vi "Main.vi"(8 "error in":errorcluster, 11 "Registration in":refnum<class "Registration.lvclass">) -> (0 "error out":errorcluster, 3 "Registration out":refnum<class "Registration.lvclass">)   [LabVIEW 2023, in "Registration.lvclass"]
doc: "The <b>Queued Message Handler</b> of the Worker that owns this VI."
uses:
  Registration.lvclass
  C:/Program Files/National Instruments/LabVIEW 2023/vi.lib/addons/_Workers/Library/Classes/Worker/Worker.lvclass
  rqp_Data.ctl
  Initialization Data.ctl
  Response Cases.ctl
  Registration.lvclass/Registration.ctl
  rql_Set File Path.ctl
  rqp_Start.ctl
  <vilib>/Utility/sysdir.llb/System Directory Type.ctl
  <vilib>/addons/_Workers/Library/Case Label.ctl
  rqp_Timeout.ctl
  <vilib>/Utility/file.llb/Write Delimited Spreadsheet (string).vi
  <vilib>/Utility/error.llb/Error Cluster From Error Code.vi
  <vilib>/addons/_Workers/Library/Classes/Message Queue/Message Queue.lvclass
  <vilib>/ErrorRing/Error Ring.xnode
  <vilib>/addons/_Workers/Library/Workers.lvlib
  Work Planer/Work Planer.lvclass
  C:/Program Files/National Instruments/LabVIEW 2023/vi.lib/addons/_Workers/Library/Classes/Workers Object/Workers Object.lvclass
  J:/Work/Cortech/KTM 1001/Workers/Registration Worker/Registration.lvclass
panel:
  in  "Period, s":u32 caption="Период регистрации, сек"
  in  "set_path":bool
  in  "open_F":bool
  in  "Registr start":bool
  out "file_path":string caption="Файл регистрации"
  out "Таймаут":u32
  out "Data":T1 {"Уд. сопротивление" format="%#.3f"; "Сопротивление" format="%#.3f"; "Диаметр" format="%#.3f"; "Длина" format="%#.3f"}
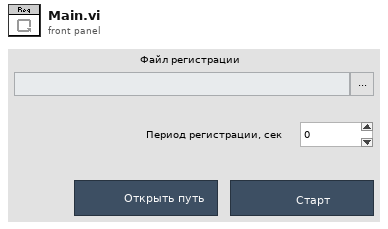
[diagram p1: front panel]
types:
  T1 = typedef "Registration.lvclass/rqp_Data.ctl" = cluster{"Дата":string, "Время":string, "Длина":dbl, "Диаметр":dbl, "Сопротивление":dbl, "Уд. сопротивление":dbl}
  T2 = typedef "Registration.lvclass/rql_Set File Path.ctl" = cluster{"String":string}
  T3 = enum8{"Enabled", "Disabled", "Disabled and Grayed Out"}
  T4 = typedef "Registration.lvclass/rqp_Start.ctl" = cluster{"Start":bool}
  T5 = typedef "Registration.lvclass/rqp_Timeout.ctl" = cluster{"Таймаут":u32}
  T6 = typedef "Registration.lvclass/Initialization Data.ctl" = cluster{"Response Cases":T7}
  T7 = typedef "Registration.lvclass/Response Cases.ctl" = cluster{"Placeholder - Can be deleted":string}
  T8 = typedef "Workers.lvlib/Case Label.ctl" = string
  T9 = typedef "System Directory Type.ctl" = i32
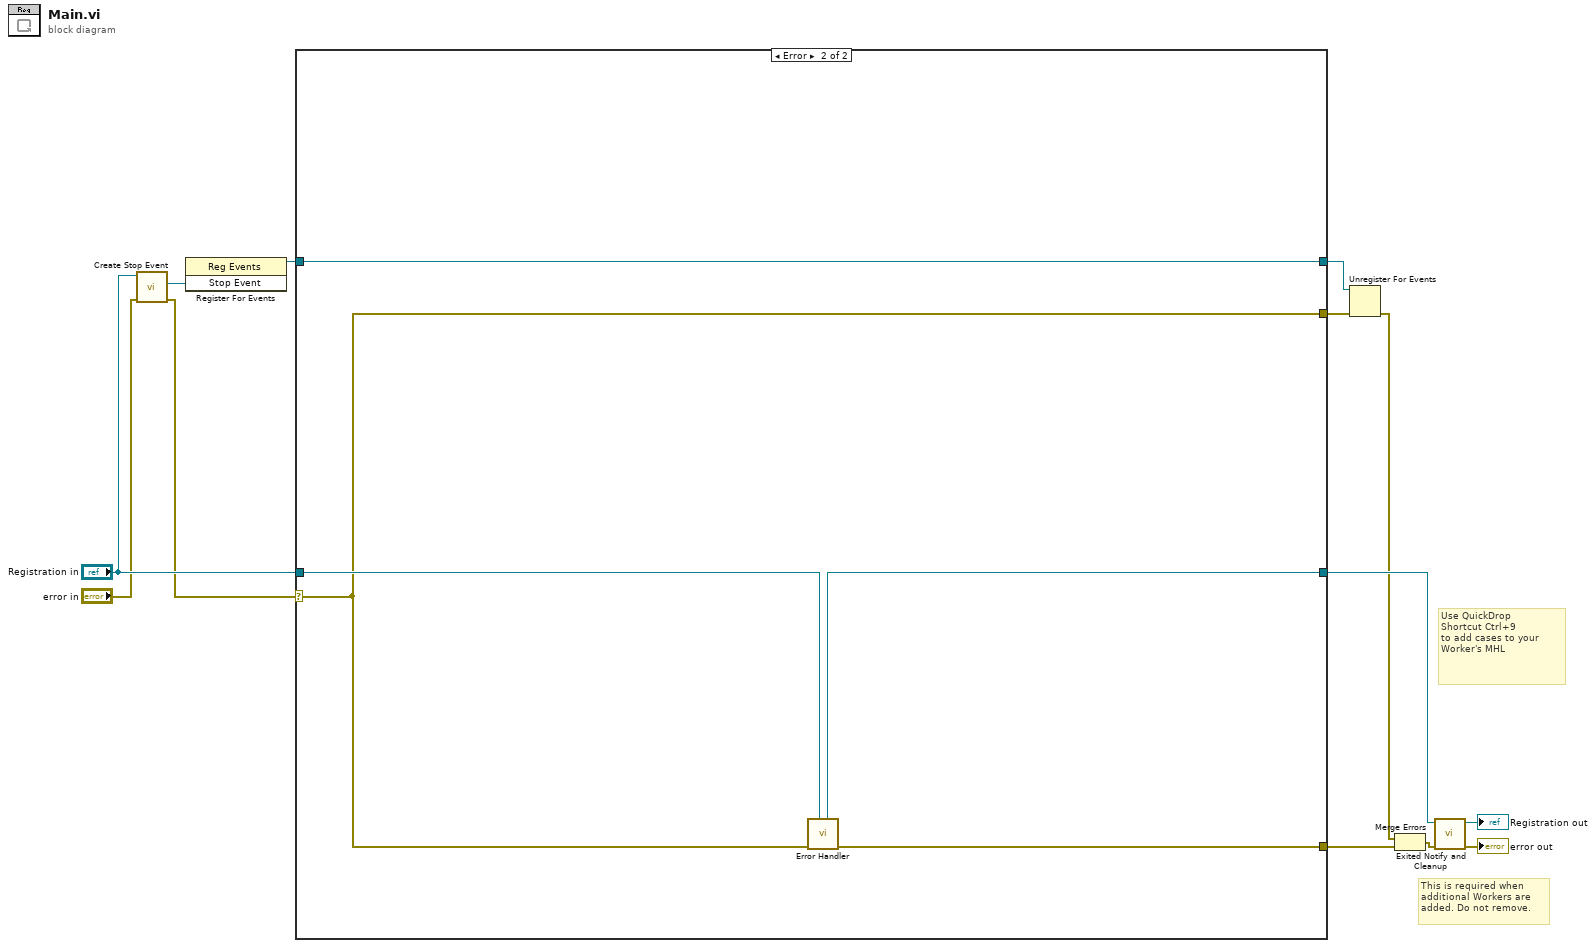
[diagram p0: block diagram]
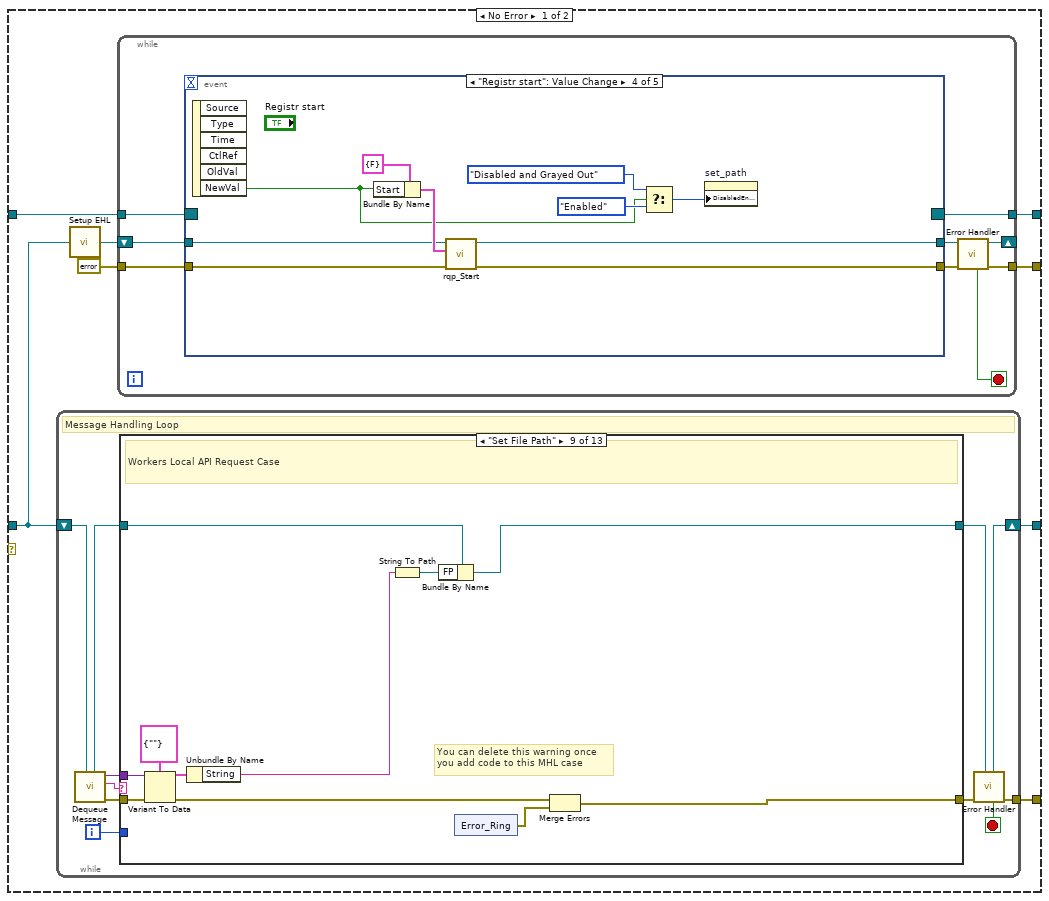
[diagram p2: hidden frame]
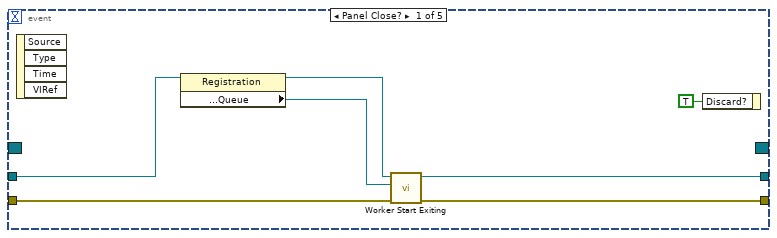
[diagram p3: hidden frame]
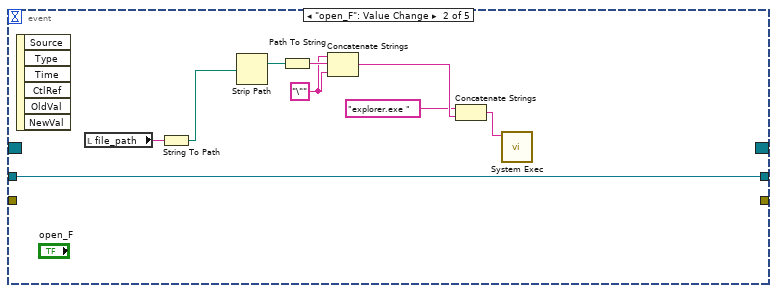
[diagram p4: hidden frame]
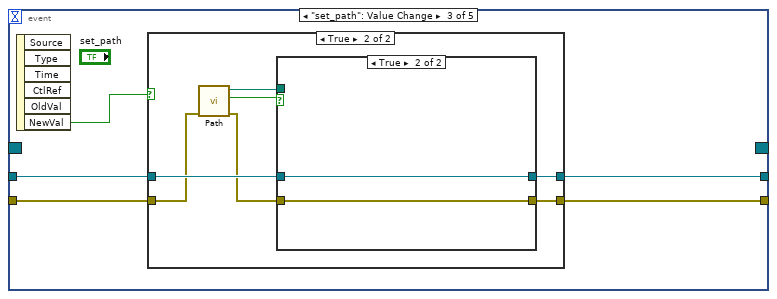
[diagram p5: hidden frame]
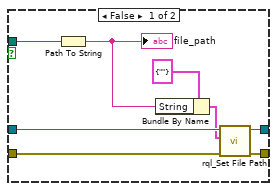
[diagram p7: hidden frame]
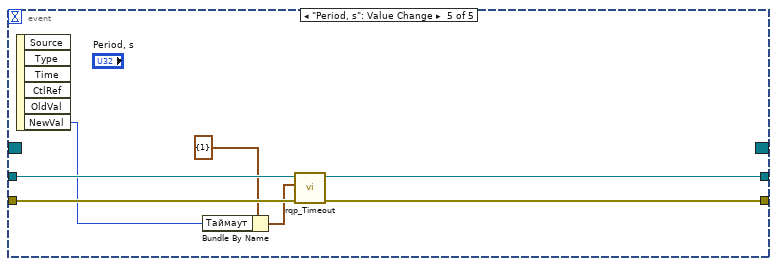
[diagram p8: hidden frame]
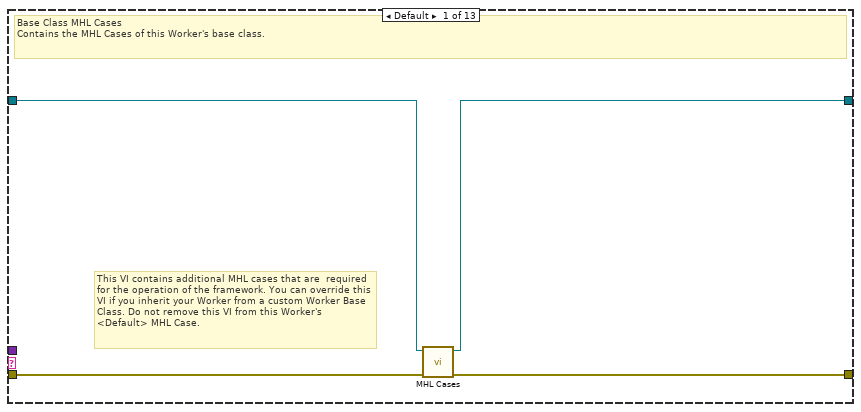
[diagram p9: hidden frame]
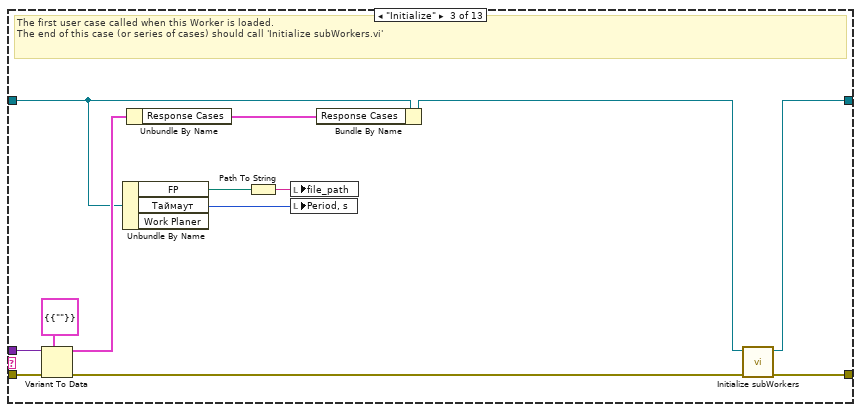
[diagram p11: hidden frame]
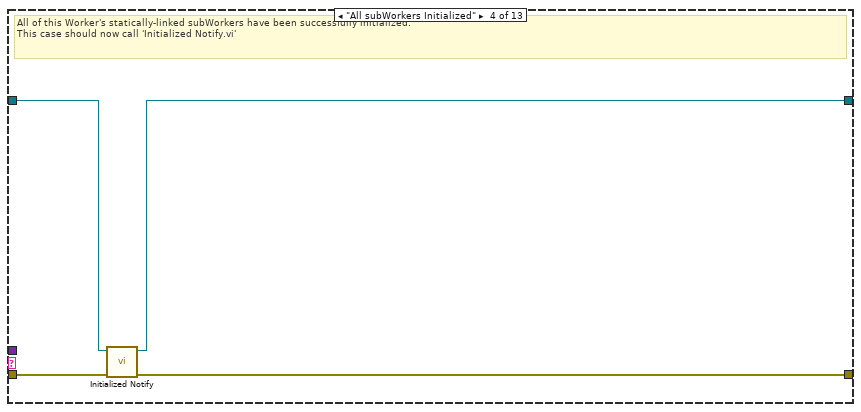
[diagram p12: hidden frame]
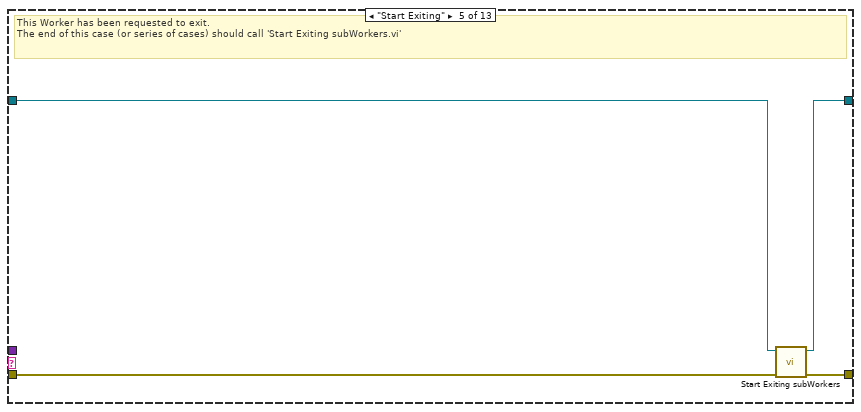
[diagram p13: hidden frame]
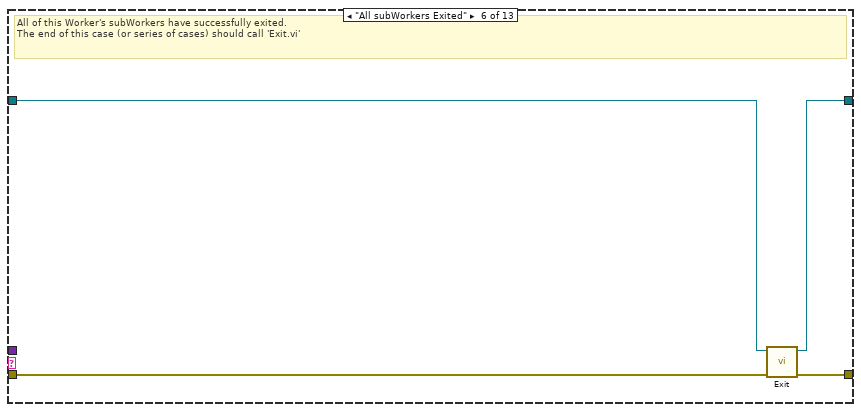
[diagram p14: hidden frame]
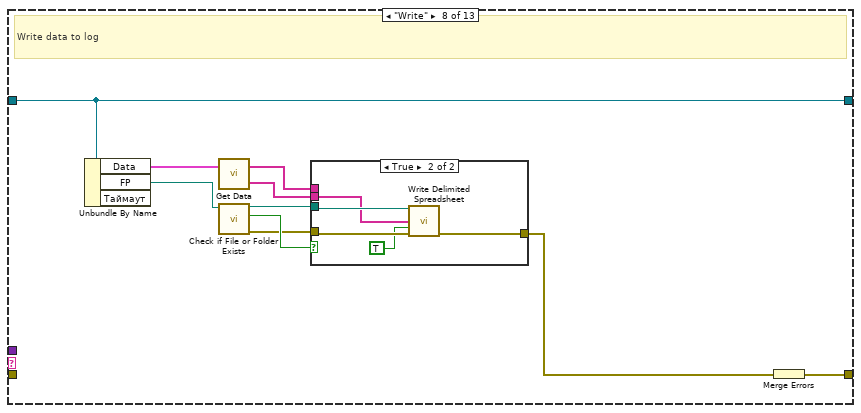
[diagram p16: hidden frame]
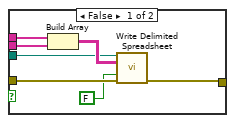
[diagram p17: hidden frame]
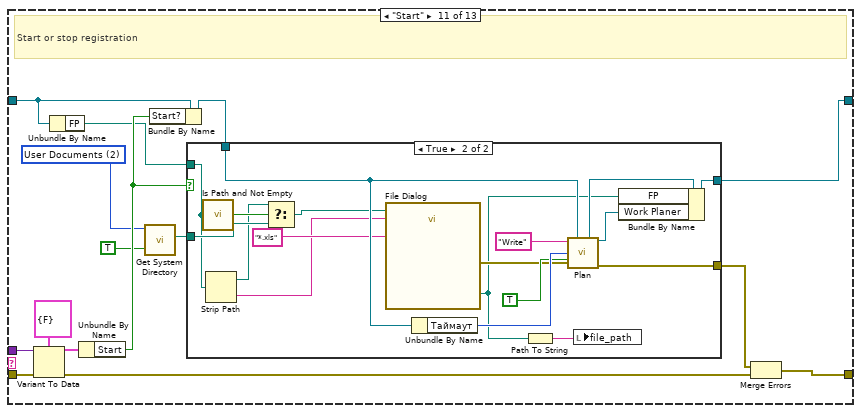
[diagram p19: hidden frame]
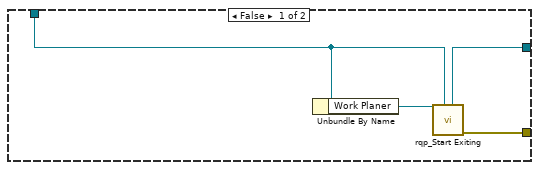
[diagram p20: hidden frame]
diagram:
  # "Use QuickDrop\nShortcut Ctrl+9\nto add cases to your\nWorker's MHL"
  # "This is required when additional Workers are added. Do not remove."
  n1 = call-dynamic "Create Stop Event.vi"("error in"="error in", "Worker"="Registration in") -> ("error out"=w5:errorcluster, "Stop Event"=w7:refnum<user-event>)  [unwired: 7 in, 1 out]
  n2 = register-events(w7) -> (reference out=w4:refnum<event-registration>)  [unwired: 2 in, 1 out]
  n3 = case shown="Error" w5 {
    tunnel: "Registration in" -> [w19 w234]
    tunnel: [w21 w235] -> w12
    tunnel: [w20 w233] -> w13
    selector: w5 -> [_ w231]
    tunnel: w4 -> [w18 w232]
    tunnel: [w15 w231] -> w3
    tunnel: [w14 w232] -> w2
    frame No Error {
      n4 = while {
        shift-right: [w96] -> w20
        shift-left: w19 -> [w98]
        tunnel: [w97] -> w21
        i -> [w89]
        stop <- w90 stop-if-true
        # "Message Handling Loop"
        n5 = call-dynamic "Dequeue Message.vi"("Worker"=w98) -> ("error out"=w95:errorcluster, "Case out"=w91:string, "Data out"=w88:variant, "Worker out"=w93:refnum<class "Registration.lvclass">)  [unwired: 6 in, 1 out]
        n6 = case "Worker MHL Case Structure (DO NOT CHANGE LABEL NAME)" shown="\"Set File Path\"" w91 {
          tunnel: w95 -> [w102 w103 w115 w121 w122 w129 w131 _ w164 w171 w186 w220 w229]
          tunnel: [w101 w103 w117 w120 w125 w128 w131 w141 w159 w171 w181 w216 w224] -> w94
          tunnel: w93 -> [w100 w104 w108 w119 w123 w127 w130 w132 w157 w170 w173 w221 w230]
          tunnel: [w99 w104 w116 w118 w124 w126 w130 w132 w155 w170 w177 w215 w223] -> w92
          tunnel: w89 -> [_ _ _ _ _ _ _ _ _ _ _ _ _]
          tunnel: w88 -> [_ _ w113 _ _ _ _ _ w161 _ w183 w217 w226]
          frame Default {
            # "This VI contains additional MHL cases that are  required for the operation of the framework. You can override this VI if you inherit your Worker from a custom Worker Base Class. Do not remove this VI from this Worker's <Default> MHL Case."
            # "Base Class MHL Cases\nContains the MHL Cases of this Worker's base class."
            n7 = call-dynamic "MHL Cases.vi"("error in"=w102, "Worker in"=w100) -> ("error out"=w101:errorcluster, "Worker out"=w99:refnum<class "Registration.lvclass">)  [unwired: 8 in]
          }
          frame "------------ FRAMEWORK CASES -----------" {
            # "Start of Workers Framework Cases"
          }
          frame "Initialize" {
            # "The first user case called when this Worker is loaded.\nThe end of this case (or series of cases) should call 'Initialize subWorkers.vi'"
            n8 = Variant To Data(error in=w115, type=T6 {"Response Cases"={"Placeholder - Can be deleted"=""}} ("Cluster"), Variant=w113) -> (data=w111:T6, error out=w114:errorcluster)
            n9 = Unbundle By Name(w108) -> ("FP"=w107:path, "Таймаут"=w105:u32)  [unwired: 1 out]
            n10 = Unbundle By Name(w111) -> ("Response Cases"=w110:T7)
            n11 = Path To String(path=w107) -> (string=w106:string)
            n12 = local write "file_path"(w106) -> ()
            n13 = local write "Period, s"(w105) -> ()
            n14 = Bundle By Name(cluster=w108, "Response Cases"=w110) -> (w112:refnum<class "Registration.lvclass">)
            n15 = call-dynamic "Initialize subWorkers.vi"("error in"=w114, "Worker"=w112) -> ("error out"=w117:errorcluster, "dup Worker out"=w116:refnum<class "Registration.lvclass">)  [unwired: 8 in]
          }
          frame "All subWorkers Initialized" {
            # "All of this Worker's statically-linked subWorkers have been successfully initialized.\nThis case should now call 'Initialized Notify.vi'"
            n16 = call-dynamic "Initialized Notify.vi"("error in"=w121, "Worker"=w119) -> ("error out"=w120:errorcluster, "dup Worker out"=w118:refnum<class "Registration.lvclass">)  [unwired: 8 in]
          }
          frame "Start Exiting" {
            # "This Worker has been requested to exit. \nThe end of this case (or series of cases) should call 'Start Exiting subWorkers.vi'"
            n17 = call-dynamic "Start Exiting subWorkers.vi"("error_in"=w122, "Worker"=w123) -> ("error out"=w125:errorcluster, "dup Worker out"=w124:refnum<class "Registration.lvclass">)  [unwired: 8 in]
          }
          frame "All subWorkers Exited" {
            # "All of this Worker's subWorkers have successfully exited. \nThe end of this case (or series of cases) should call 'Exit.vi'"
            n18 = call-dynamic "Exit.vi"("error_in"=w129, "Worker"=w127) -> ("error out"=w128:errorcluster, "dup Worker out"=w126:refnum<class "Registration.lvclass">)  [unwired: 8 in]
          }
          frame "------------- LOCAL API CASES -------------" {
            # "Start of Workers Local API Cases"
          }
          frame "Write" {
            # "Write data to log"
            n19 = Unbundle By Name(w132) -> ("Data"=w140:T1, "FP"=w139:path)  [unwired: 1 out]
            n20 = call "Get Data.vi"("Data"=w140) -> ("Array of Data"=w137:string[], "Array of Headers"=w136:string[])  [unwired: 1 in]
            n21 = call <vilib>:"Check if File or Folder Exists.vi"("path"=w139) -> ("error out"=w135:errorcluster, "file or folder exists?"=w138:bool, "dup path"=w134:path)  [unwired: 8 in]
            n22 = case shown="True" w138 {
              tunnel: w137 -> [w147 w151]
              tunnel: w136 -> [w148 _]
              tunnel: w135 -> [w145 w153]
              tunnel: w134 -> [w143 w152]
              tunnel: [w142 w149] -> w133
              frame False {
                n23 = Build Array(w148, w147) -> (w146:string[][])
                n24 = call-poly <vilib>:"Write Delimited Spreadsheet.vi"("file path (dialog if empty)"=w143, "2D data"=w146, "append to file? (new file:F)"=FALSE, "error in (no error)"=w145) -> ("error out"=w142:errorcluster)  [unwired: 10 in, 1 out]
              }
              frame True {
                n25 = call-poly <vilib>:"Write Delimited Spreadsheet.vi"("file path (dialog if empty)"=w152, "1D data"=w151, "append to file? (new file:F)"=TRUE, "error in (no error)"=w153) -> ("error out"=w149:errorcluster)  [unwired: 10 in, 1 out]
              }
            }
            n26 = Merge Errors(w133) -> (w141:errorcluster)
          }
          frame "Set File Path" {
            # "You can delete this warning once\nyou add code to this MHL case"
            # "Workers Local API Request Case"
            n27 = Variant To Data(error in=w164, type=T2 {"String"=""} ("Data"), Variant=w161) -> (data=w160:T2, error out=w163:errorcluster)
            n28 = Unbundle By Name(w160) -> ("String"=w154:string)
            n29 = String To Path(string=w154) -> (path=w156:path)
            n30 = Bundle By Name(cluster=w157, "FP"=w156) -> (w155:refnum<class "Registration.lvclass">)
            n31 = xnode ("Error_Ring")() -> ("error out"=w158:errorcluster)
            n32 = Merge Errors(w163, w158) -> (w159:errorcluster)
          }
          frame "------------- PUBLIC API CASES -------------" {
            # "Start of Workers Public API Cases"
          }
          frame "Start" {
            w175 = T9 2 items=["User Home"=0, "User Desktop"=1, "User Documents"=2, "User Application Data"=3, "User Preferences"=4, "User Temporary"=5, "Public Documents"=6, "Public Application Data"=7, "Public Preferences"=8, "Public Cache"=13, "System Core Libraries"=9, "System Installed Libraries"=10, "Application Files"=11, "Boot Volume Root"=12] ("system directory type")
            # "Start or stop registration"
            n33 = Variant To Data(error in=w186, type=T4 {"Start"=FALSE} ("Data"), Variant=w183) -> (data=w182:T4, error out=w185:errorcluster)
            n34 = Unbundle By Name(w173) -> ("FP"=w172:path)
            n35 = Unbundle By Name(w182) -> ("Start"=w180:bool)
            n36 = call <vilib>:"Get System Directory.vi"("create directory if not found? (F)"=TRUE, "system directory type"=w175) -> ("system directory"=w174:path)  [unwired: 9 in]
            n37 = Bundle By Name(cluster=w173, "Start?"=w180) -> (w178:refnum<class "Registration.lvclass">)
            n38 = case shown="True" w180 {
              tunnel: [w190 w201] -> w179
              tunnel: w178 -> [w189 w205]
              tunnel: [w187 w203] -> w177
              tunnel: w174 -> [_ w198]
              tunnel: w172 -> [_ w197]
              frame False {
                n39 = Unbundle By Name(w189) -> ("Work Planer"=w188:refnum<class "Work Planer.lvclass">)
                n40 = call "rqp_Start Exiting.vi"("Caller in"=w189, "Work Planer in"=w188) -> ("error out"=w190:errorcluster, "dup Caller out"=w187:refnum<class "Registration.lvclass">)  [unwired: 7 in, 1 out]
              }
              frame True {
                n41 = call <vilib>:"Is Path and Not Empty.vi"("path"=w197) -> ("Is Path and Not Empty?"=w199:bool)  [unwired: 4 in]
                n42 = Strip Path(path=w197) -> (stripped path=w196:path, name=w193:string)
                n43 = Select(t=w196, s=w199, f=w198) -> (s? t:f=w194:path)
                n44 = call "File Dialog"("start path"=w194, "default name"=w193, "pattern (all files)"="*.xls") -> ("selected path"=w191:path, "error out"=w202:errorcluster)  [unwired: 9 in, 2 out]
                n45 = Unbundle By Name(w205) -> ("Таймаут"=w207:u32)
                n46 = Path To String(path=w191) -> (string=w192:string)
                n47 = call "Plan.vi"("Response Case"=T8 "Write" ("Case Label"), "Caller in"=w205, "Timeout (1000ms)"=w207, "Continius? (F)"=TRUE, "error in (no error)"=w202) -> ("dup Caller out"=w204:refnum<class "Registration.lvclass">, "Work Planer out"=w200:refnum<class "Work Planer.lvclass">, "error out"=w201:errorcluster)  [unwired: 8 in]
                n48 = local write "file_path"(w192) -> ()
                n49 = Bundle By Name(cluster=w204, "FP"=w191, "Work Planer"=w200) -> (w203:refnum<class "Registration.lvclass">)
              }
            }
            n50 = Merge Errors(w179, w185) -> (w181:errorcluster)
          }
          frame "Data" {
            # "Data for registration"
            n51 = Variant To Data(error in=w220, type=T1 {"Дата"="", "Время"="", "Длина"=0.0, "Диаметр"=0.0, "Сопротивление"=0.0, "Уд. сопротивление"=0.0} ("Data"), Variant=w217) -> (data=w214:T1, error out=w219:errorcluster)
            n52 = Get Date/Time In Seconds() -> (seconds since 1Jan1904=w210:timestamp)
            n53 = Get Date/Time String(seconds (now)=w210, want seconds? (F)=TRUE) -> (date string=w212:string, time string=w213:string)  [unwired: 1 in]
            n54 = Bundle By Name(cluster=w214, "Дата"=w212, "Время"=w213) -> (w209:T1)
            "Data" <- w209
            n55 = Bundle By Name(cluster=w221, "Data"=w209) -> (w215:refnum<class "Registration.lvclass">)
            n56 = Merge Errors(w219) -> (w216:errorcluster)
          }
          frame "Timeout" {
            # "Set new timeout registration"
            n57 = Variant To Data(error in=w229, type=T5 {"Таймаут"=1} ("Data"), Variant=w226) -> (data=w225:T5, error out=w228:errorcluster)
            n58 = Unbundle By Name(w225) -> ("Таймаут"=w222:u32)
            "Таймаут" <- w222
            n59 = Bundle By Name(cluster=w230, "Таймаут"=w222) -> (w223:refnum<class "Registration.lvclass">)
            n60 = Merge Errors(w228) -> (w224:errorcluster)
          }
        }
        n61 = call-dynamic "Error Handler.vi"("Worker"=w92, "error_in"=w94) -> ("error out"=w97:errorcluster, "Stop Loop"=w90:bool, "Worker out"=w96:refnum<class "Registration.lvclass">)  [unwired: 7 in]
      }
      n62 = call-dynamic "Setup EHL.vi"("Worker"=w19) -> ("Worker out"=w17:refnum<class "Registration.lvclass">)  [unwired: 14 in]
      n63 = while {
        tunnel: w18 -> [w30]
        shift-right: [w25] -> _
        shift-left: w17 -> [w29]
        tunnel: errorcluster {"status"=FALSE, "code"=0, "source"=""} ("error_in") -> [w28]
        tunnel: [w23] -> w15
        tunnel: [w22] -> w14
        stop <- w24 stop-if-true
        n64 = event shown="[3] \"Registr start\": Value Change" {
          selector: w30 -> [_ _ _ _ _]
          dyn-events: [_ _ _ _ _] -> w22
          timeout: _ -> [_ _ _ _ _]
          tunnel: w29 -> [w35 w46 w50 w78 w87]
          tunnel: [w34 w46 w49 w75 w86] -> w27
          tunnel: [w32 _ w47 w76 w84] -> w26
          tunnel: w28 -> [w31 _ w48 w77 w85]
          event Panel Close? {
            n65 = event-data() -> ()  [unwired: 1 in, 4 out]
            n66 = property class="Registration"(reference=w35) -> (reference out=w37:refnum<class "Registration.lvclass">, "Accessors:Read:Public API:Queue"=w36:refnum<class "Message Queue.lvclass">)  [unwired: 1 in, 1 out]
            n67 = call-dynamic "Worker Start Exiting.vi"("error_in"=w31, "Message Queue"=w36, "Worker"=w37) -> ("error out"=w32:errorcluster, "dup Worker out"=w34:refnum<class "Registration.lvclass">)  [unwired: 7 in]
            n68 = event-data("Discard?"=TRUE) -> ()  [unwired: 1 in, 1 out]
          }
          event "open_F": Value Change {
            w40 = "\""
            n69 = event-data() -> ()  [unwired: 1 in, 6 out]
            n70 = local read "file_path"() -> (w39:string)
            n71 = String To Path(string=w39) -> (path=w38:path)
            n72 = Strip Path(path=w38) -> (stripped path=w45:path)  [unwired: 1 out]
            n73 = Path To String(path=w45) -> (string=w43:string)
            n74 = Concatenate Strings(w40, w43, w40) -> (w44:string)
            n75 = Concatenate Strings("explorer.exe " ("command line"), w44) -> (w42:string)
            n76 = call <vilib>:"System Exec.vi"("command line"=w42) -> ()  [unwired: 7 in, 4 out]
          }
          event "set_path": Value Change {
            n77 = event-data() -> ("NewVal"=w51:bool)  [unwired: 1 in, 5 out]
            n78 = case shown="True" w51 {
              tunnel: w50 -> [w53 w58]
              tunnel: [w53 w57] -> w49
              tunnel: w48 -> [w52 w56]
              tunnel: [w52 w54] -> w47
              frame False {
              }
              frame True {
                n79 = call "Path.vi"("error in"=w56) -> ("error out"=w55:errorcluster, "Cancelled"=w60:bool, "Selected Path"=w59:path)  [unwired: 8 in]
                n80 = case shown="True" w60 {
                  tunnel: w59 -> [w68 _]
                  tunnel: w58 -> [w67 w70]
                  tunnel: [w66 w70] -> w57
                  tunnel: w55 -> [w65 w69]
                  tunnel: [w64 w69] -> w54
                  frame False {
                    n81 = Path To String(path=w68) -> (string=w61:string)
                    "file_path" <- w61
                    n82 = Bundle By Name(cluster=T2 {"String"=""} ("Data in"), "String"=w61) -> (w62:T2)
                    n83 = call "rql_Set File Path.vi"("error in"=w65, "Data in"=w62, "Registration in"=w67) -> ("error out"=w64:errorcluster, "dup Registration out"=w66:refnum<class "Registration.lvclass">)  [unwired: 7 in]
                  }
                  frame True {
                  }
                }
              }
            }
          }
          event "Registr start": Value Change {
            n84 = event-data() -> ("NewVal"=w71:bool)  [unwired: 1 in, 5 out]
            n85 = Bundle By Name(cluster=T4 {"Start"=FALSE} ("Data in"), "Start"=w71) -> (w79:T4)
            n86 = call "rqp_Start.vi"("error in"=w77, "Data in"=w79, "Registration in"=w78) -> ("error out"=w76:errorcluster, "dup Registration out"=w75:refnum<class "Registration.lvclass">)  [unwired: 6 in, 1 out]
            n87 = Select(t=T3."Disabled and Grayed Out" ("Disabled"), s=w71, f=T3."Enabled" ("Disabled")) -> (s? t:f=w72:T3)
            n88 = property on="set_path" class="Bool"("DisabledEnum"=w72) -> ()  [unwired: 2 in, 2 out]
          }
          event "Period, s": Value Change {
            n89 = event-data() -> ("NewVal"=w82:u32)  [unwired: 1 in, 5 out]
            n90 = Bundle By Name(cluster=T5 {"Таймаут"=1} ("Data in"), "Таймаут"=w82) -> (w81:T5)
            n91 = call "rqp_Timeout.vi"("error in"=w85, "Data in"=w81, "Registration in"=w87) -> ("error out"=w84:errorcluster, "dup Registration out"=w86:refnum<class "Registration.lvclass">)  [unwired: 6 in, 1 out]
          }
        }
        n92 = call-dynamic "Error Handler.vi"("Worker"=w27, "error_in"=w26) -> ("error out"=w23:errorcluster, "Stop Loop"=w24:bool, "Worker out"=w25:refnum<class "Registration.lvclass">)  [unwired: 7 in]
      }
    }
    frame Error {
      n93 = call-dynamic "Error Handler.vi"("Worker"=w234, "error_in"=w231) -> ("error out"=w235:errorcluster, "Worker out"=w233:refnum<class "Registration.lvclass">)  [unwired: 7 in, 1 out]
    }
  }
  n94 = Unregister For Events(event registration refnum=w2, error in=w3) -> (error out=w1:errorcluster)
  n95 = Merge Errors(w1, w12) -> (w9:errorcluster)
  n96 = call-dynamic "Exited Notify and Cleanup.vi"("error_in"=w9, "Worker"=w13) -> ("error out"=→"error out":errorcluster, "dup Worker out"=→"Registration out":refnum<class "Registration.lvclass">)  [unwired: 8 in]
